vi "Routing and Faulting Hardware API Constants.vi"() -> ()   [LabVIEW 2020, in "Routing and Faulting Hardware API.lvlib"]
uses:
  Routing and Faulting Hardware API.lvlib
panel:
  in  "Tab Control":enum32{"Properties", "GUID"}(tab)
  in  "Properties:Initially Connected Endpoints":string="Routing and Faulting.Initially Connected Endpoints"
  in  "Properties:Configuration Revision":string="Routing and Faulting.Configuration Revision"
  in  "Properties:Possible Connections":string="Routing and Faulting.Possible Connections"
  in  "Properties:Addressable Endpoints":string="Routing and Faulting.Addressable Endpoints"
  in  "Properties:API Version":string="Routing and Faulting.API Version"
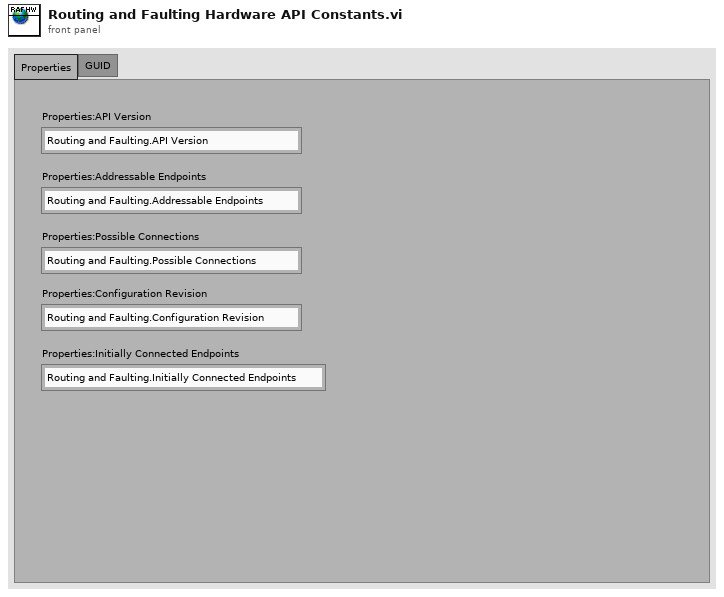
[diagram p1: front panel]
diagram:
